vi "Yokogawa.vi"(8 "error in (no error)":errorcluster, 11 "Generic Instrument.lvlib:Generic Instrument.lvclass":refnum<class "Generic Instrument.lvclass">) -> (0 "error out":errorcluster, 2 "String Contains?":bool, 3 "Generic Instrument.lvlib:Generic Instrument.lvclass 2":refnum<class "Generic Instrument.lvclass">)   [LabVIEW 2014, in "Generic Instrument.lvlib" / "Generic Instrument.lvclass"]
uses:
  Generic Instrument.lvclass
  Generic Instrument.lvclass/Generic Instrument.ctl
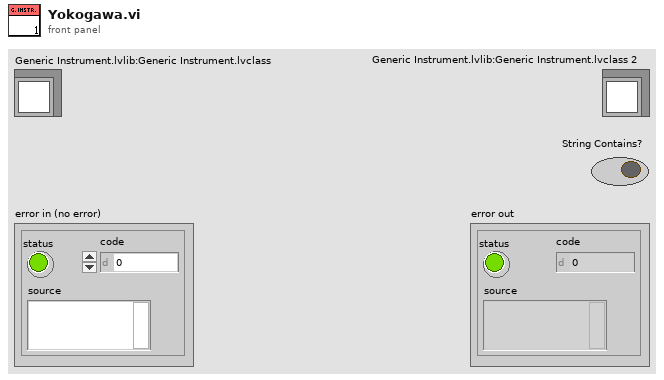
[diagram p1: front panel]
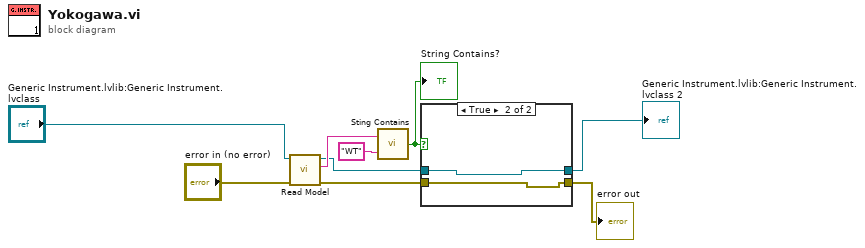
[diagram p0: block diagram]
diagram:
  n1 = call "Read Model.vi"("error in (no error)"="error in (no error)", "Generic Instrument in"="Generic Instrument.lvlib:Generic Instrument.lvclass") -> ("error out"=w3:errorcluster, "Model"=w7:string, "Generic Instrument out"=w4:refnum<class "Generic Instrument.lvclass">)  [unwired: 7 in]
  n2 = call "Sting Contains.vi"("Expression to evaluate"="WT", "Input String"=w7) -> ("Boolean"=w5:bool)
  "String Contains?" <- w5
  n3 = case shown="True" w5 {
    tunnel: w4 -> [w11 w13]
    tunnel: w3 -> [w10 w12]
    tunnel: [w11 w13] -> w1
    tunnel: [w10 w12] -> w2
    frame False {
    }
    frame True {
    }
  }
  "Generic Instrument.lvlib:Generic Instrument.lvclass 2" <- w1
  "error out" <- w2
